vi "Acquire Data using 5772 without DRAM_sim2.vi"() -> ()   [LabVIEW 2011]
uses:
  <vilib>/Platform/TimedLoop/XDataNode/timing_clust.ctl
  <vilib>/Platform/TimedLoop/XDataNode/nitl_modes.ctl
  <vilib>/Platform/TimedLoop/XDataNode/wakeup.ctl
  <instrlib>/FlexRIO/Libraries/Acquisition Engine/FPGA/Implementation/Pack 8-I16 As U128.vi
  <instrlib>/FlexRIO/Libraries/Host Transfer/FPGA/Implementation/Write to Host-Bound Domain (128-bit to 64-bit).vi
  <vilib>/rvi/FIFO/Fifo_Resource/nirvififoEmulationSetSize.vi
  <vilib>/rvi/DataTransferAndStorage/Container/Common/niFpgaContainerGetUniqueNameForEmu.vi
  Channel Data/Data from Channel 0 and Channel 1.vi
  <instrlib>/FlexRIO/Libraries/Acquisition Engine/FPGA/Implementation/acqEngineNRecordStateMachine.vi
  <vilib>/Platform/TimedLoop/XDataNode/XDataNode.xnode
  <vilib>/rvi/DataTransferAndStorage/Container/XNode/niFpgaContainer.xnode
  <vilib>/rvi/FIFO/Fifo_Resource/nirvififoEmulationRead.vi
  <vilib>/rvi/FXPMathLib/basic elements/FxpDiscreteDelay/XNode/nifxpmath_DiscreteDelay.xnode
  <vilib>/rvi/FIFO/Fifo_Resource/nirvififoEmulationWrite.vi
  <vilib>/Platform/TimedLoop/XDataNode/XDNodeRunTimeDep.lvlib
  <vilib>/eio/EIONode/EIONode.xnode
  <instrlib>/FlexRIO/Libraries/Host Transfer/Host Transfer.lvlib
  <instrlib>/FlexRIO/Libraries/Acquisition Engine/Acquisition Engine.lvlib
  <vilib>/rvi/eio/common/nirviEmuTemplateMethod_errors.vi
panel:
  out "Trig[N-3]":bool
  out "Trig[N-2]":bool
  out "Trig[N-1]":bool
  out "Trig[N]":bool
  out "Q3":i16[](array[numeric])
  out "Q2":i16[](array[numeric])
  out "Q1":i16[](array[numeric])
  out "Channel 1":i16(graph)
  out "Channel 0":i16(graph)
  out "NumSamplestoHost":u32
  out "NumSamplesAcquired":u32
  out "Host FIFO Timed Out?":bool
  in  "Host Trigger":bool=TRUE
  in  "Trigger Type":T1(ring)=enum."Software Trigger"
  out "IO Module\\Initialization Done":bool
  in  "acq.Post Trig":u32=10
  in  "acq.Pre Trig":u32=2 min=2 step=1
  in  "acq.Record Count":u32=1
  in  "acq.Initiate":bool=TRUE
  # "Digitial Trigger Input:\nPXI_Trig0 or DIO 0 on CB Front Panel"
  # "Interactive Mode Instructions\n1) Run the Emulation Mode VI for Stimulus\n1) Click on acq.Initiate, First to False and Then to True\n2) Click on Host Trigger"
  # "Trigger Selection"
  # "Acquisition Engine"
  # "Status"
  # "Record Retrieval"
  # "Memory Configuration"
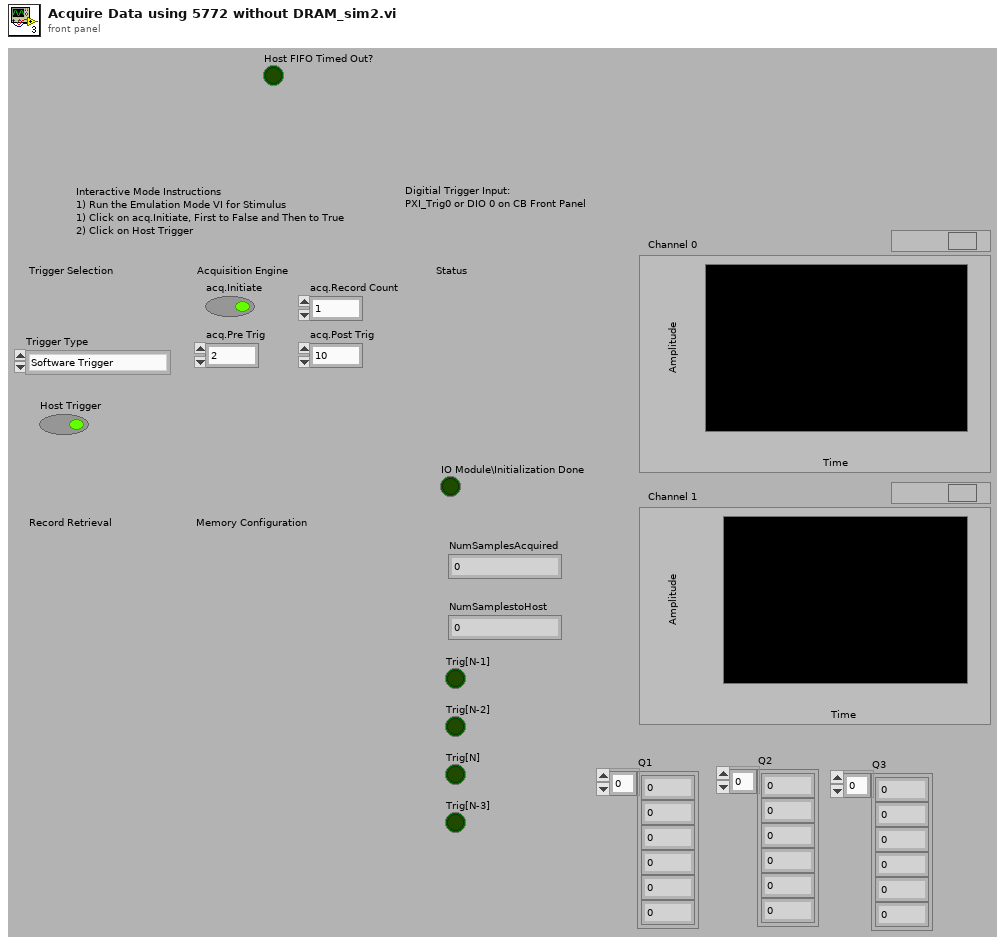
[diagram p1: front panel]
types:
  T1 = enum8{"Immediate Trigger", "Software Trigger", "External Digital Trigger", "Analog Trigger"}
  T2 = typedef "XDNodeRunTimeDep.lvlib/timing_clust.ctl" = cluster{"Expected End [f-1]":u64, "Actual End [f-1]":u64, "Finished Late? [f-1]":bool, "Expected End [i-1]":u64, "Actual End [i-1]":u64, "Finished Late? [i-1]":bool, "Expected Start [i]":u64, "Actual Start [i]":u64, "Expected Start [f]":u64, "Actual Start [f]":u64, "Source Name":string, "Structure Name":string, "Period":i64, "Deadline":i64, "Offset":i64, "Start":i64, "Priority":i32, "Timeout":i32, "Mode":T3, "Wakeup Reason":T4, "Error":errorcluster, "Source Type":string, "Secondary Source Type":string, "Global End Time":u64, "Global Start Time":u64, "Frame Duration":u64, "Iteration Duration":u64, "Assigned CPU":i32, "I/O Scan Engine Mode":u32}
  T3 = typedef "XDNodeRunTimeDep.lvlib/nitl_modes.ctl" = enum32{"No Change", "Process missed periods, maintain original phase", "Discard missed periods, maintain original phase", "Process missed periods, ignore original phase", "Discard missed periods, ignore original phase"}
  T4 = typedef "XDNodeRunTimeDep.lvlib/wakeup.ctl" = enum32{"Normal", "Aborted", "Asynchronous wakeup", "Timing source error", "Timed loop error", "Timeout"}
  T5 = typedef "acqEngineStates v1.ctl" = cluster{"Triggered":bool, "TrigArmed":bool, "RdyForArm":bool, "Reserved":bool}
  T6 = typedef "Memory.lvlib/U128.ctl" = u8[]
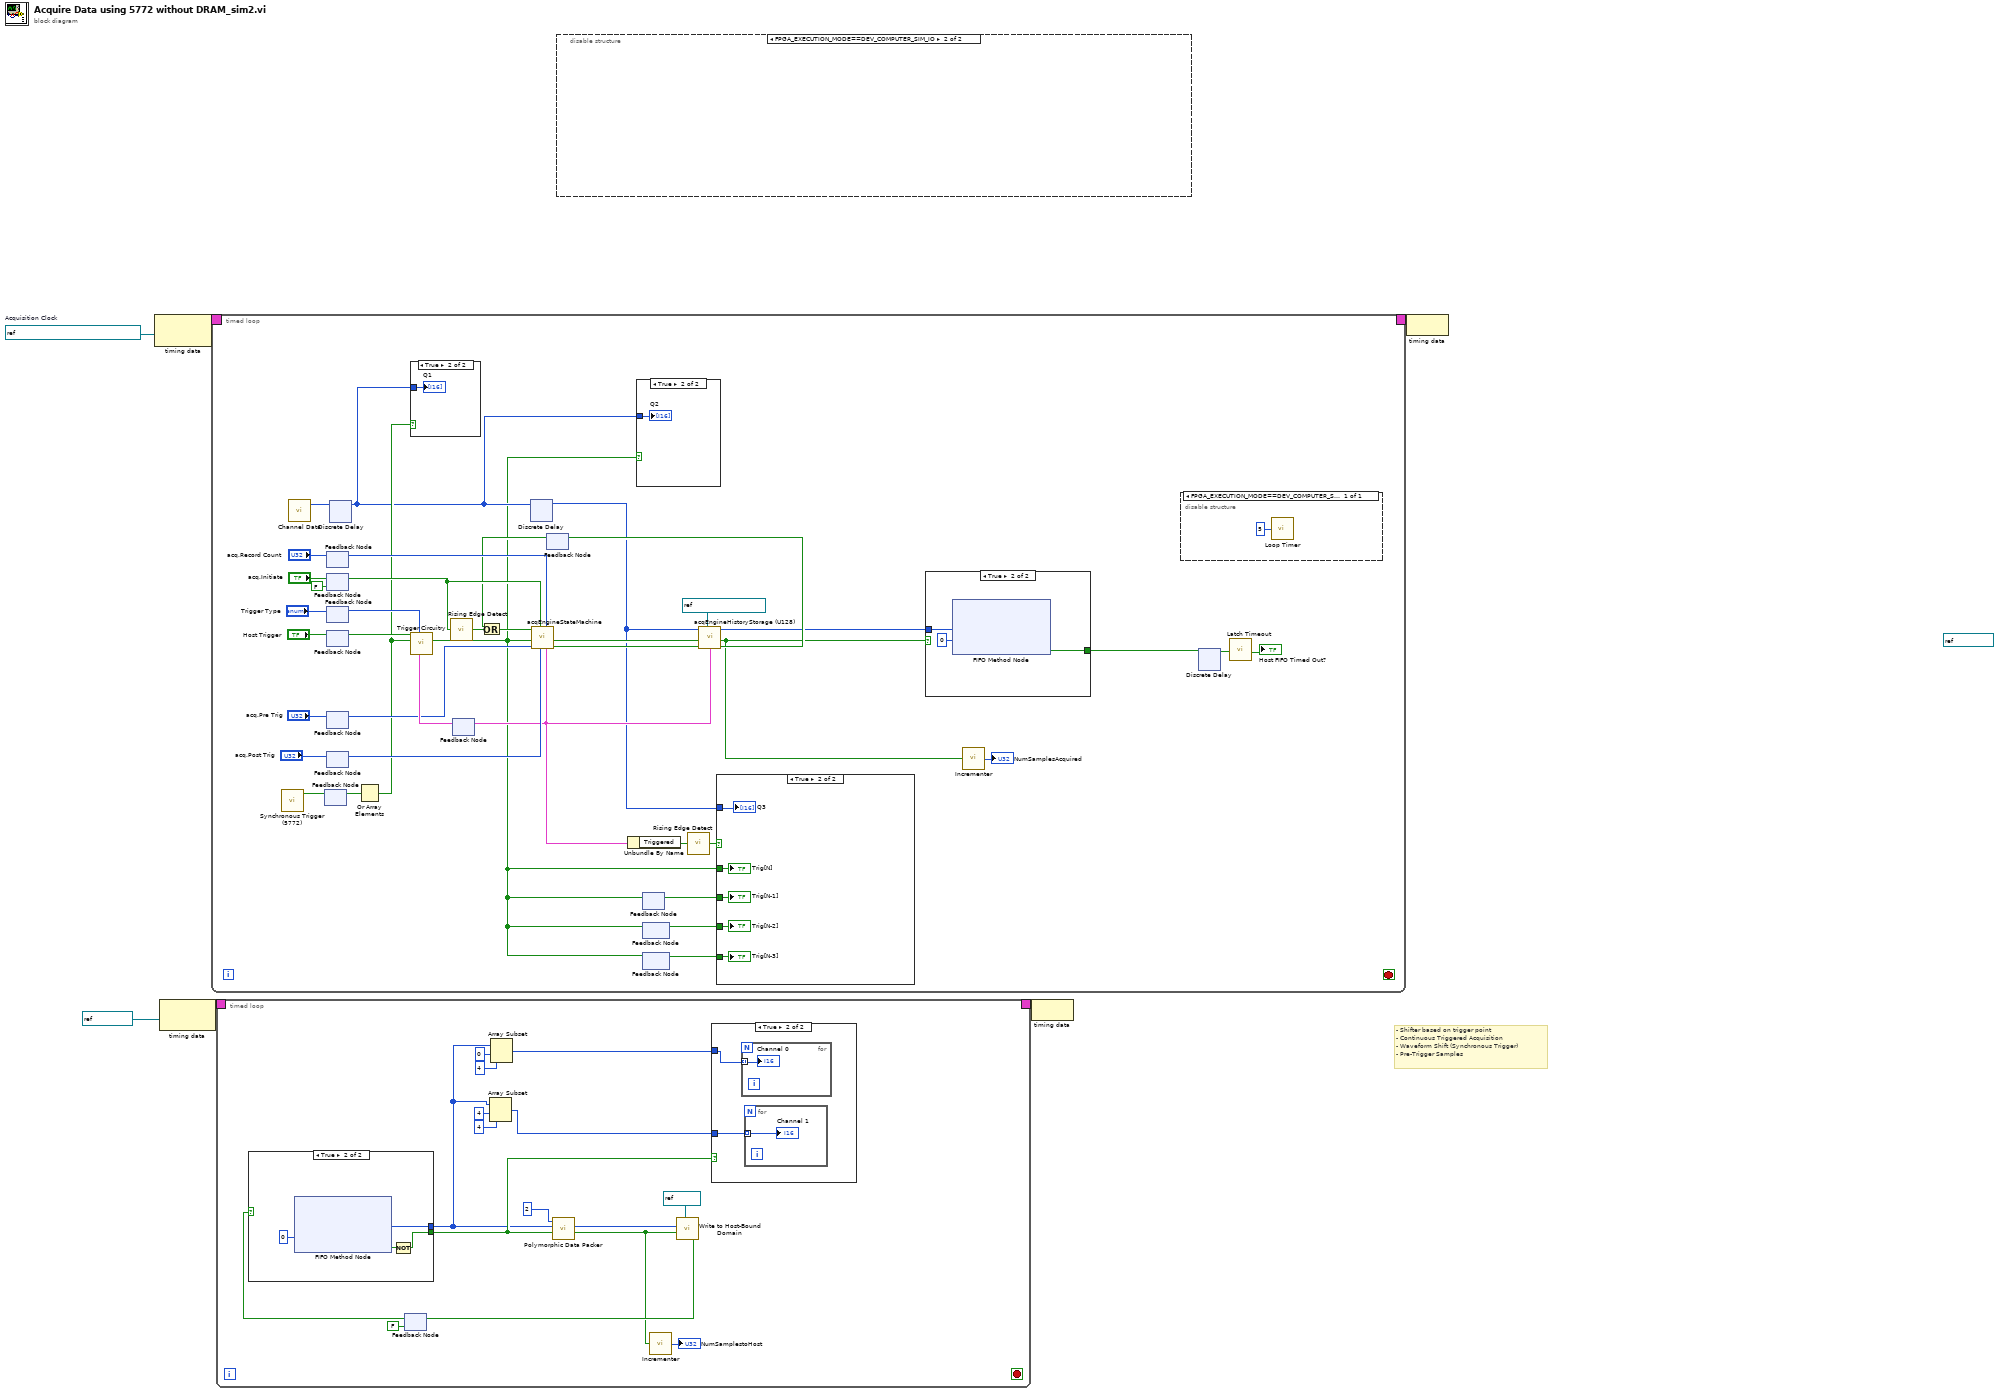
[diagram p0: block diagram]
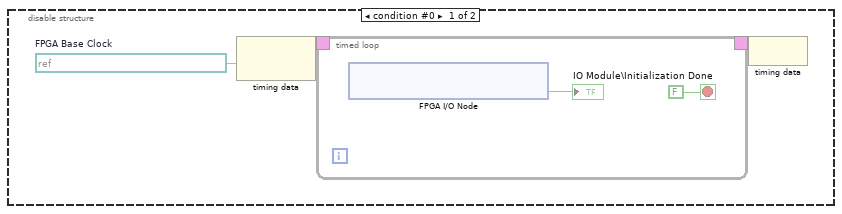
[diagram p2: hidden frame]
diagram:
  (unwired) refnum<k21> "To Host" ("FIFO In")
  w4 = refnum<k21> "IO Module Clock 0"  # Acquisition Clock
  # "- Shifter based on trigger point\n- Continuous Triggered Acquisition\n- Waveform Shift (Synchronous Trigger)\n- Pre-Trigger Samples"
  n1 = node-c288(w4) -> (w6:T2)
  n2 = node-c288(refnum<k21> "125MHz" ("Source Name")) -> (w3:T2)
  n3 = timed-loop {
    timing: w6 -> [_]
    timing-out: [_] -> w5
    stop <- _ stop-if-true
    n4 = call "Synchronous Trigger (5772).vi"() -> ("Trigger"=w22:bool[])  [unwired: 10 in, 1 out]
    n5 = call-poly "Channel Data.vi"() -> ("Channels Data"=w36:i16[])  [unwired: 11 in]
    n6 = feedback-in #1(w22) -> ()
    n7 = feedback #1() -> (w21:bool[])  [unwired: 1 in]
    n8 = feedback-in #2("acq.Record Count") -> ()
    n9 = feedback #2() -> (w40:u32)  [unwired: 1 in]
    n10 = feedback-in #3("acq.Initiate") -> ()
    n11 = feedback #3(FALSE ("acq.Initiate")) -> (w26:bool)
    n12 = feedback #4() -> (w38:T1)  [unwired: 1 in]
    n13 = feedback-in #4("Trigger Type") -> ()
    n14 = feedback-in #5("Host Trigger") -> ()
    n15 = feedback #5() -> (w37:bool)  [unwired: 1 in]
    n16 = feedback-in #6("acq.Pre Trig") -> ()
    n17 = feedback #6() -> (w35:u32)  [unwired: 1 in]
    n18 = feedback-in #7("acq.Post Trig") -> ()
    n19 = feedback #7() -> (w34:u32)  [unwired: 1 in]
    n20 = xnode "Discrete Delay"("D"=w36) -> ("Q"=w13:i16[])
    n21 = Or Array Elements(Boolean array=w21) -> (logical OR=w16:bool)
    n22 = case shown="True" w16 {
      tunnel: w13 -> [_ w53]
      frame False {
      }
      frame True {
        "Q1" <- w53
      }
    }
    n23 = call <userlib>:"Rising Edge Detect.vi"("signal"=w26) -> ("edge detected"=w23:bool)  [unwired: 14 in]
    n24 = feedback #8() -> (w42:T5)  [unwired: 1 in]
    n25 = call <userlib>:"Trigger Circuitry.vi"("State Machine State"=w42, "Trigger Type"=w38, "Digital Line Read"=w16, "Software Trigger from Host"=w37) -> ("Trigger Out"=w9:bool)  [unwired: 6 in, 1 out]
    n26 = xnode "Discrete Delay"("D"=w13) -> ("Q"=w12:i16[])
    n27 = feedback #9() -> (w24:bool)  [unwired: 1 in]
    n28 = Or(x=w24, y=w23) -> (x .or. y?=w25:bool)
    n29 = call-poly <instrlib>:"acqEngineStateMachine.vi"("acq.Record Count"=w40, "acq.Post Trig"=w34, "acq.Initiate"=w26, "acq.Pre Trig"=w35, "Trig"=w9, "StartTrig"=w25) -> ("PostTrigComplete"=w33:bool, "AcqInProgress"=w20:bool, "states"=w15:T5)  [unwired: 3 in]
    n30 = feedback-in #8(w15) -> ()
    n31 = Unbundle By Name(w15) -> ("Triggered"=w14:bool)
    n32 = case shown="True" w9 {
      tunnel: w13 -> [_ w52]
      frame False {
      }
      frame True {
        "Q2" <- w52
      }
    }
    n33 = feedback-in #10(w9) -> ()
    n34 = feedback #10() -> (w11:bool)  [unwired: 1 in]
    n35 = feedback #11() -> (w10:bool)  [unwired: 1 in]
    n36 = feedback-in #11(w9) -> ()
    n37 = feedback #12() -> (w8:bool)  [unwired: 1 in]
    n38 = feedback-in #12(w9) -> ()
    n39 = call <userlib>:"Rising Edge Detect.vi"("signal"=w14) -> ("edge detected"=w7:bool)  [unwired: 14 in]
    n40 = call "acqEngineHistoryStorage (U128).vi"("FIFO Out"=refnum<k21> "HistoryFIFOU128", "PostTrigComplete"=w33, "AcqInProgress"=w20, "states"=w15, "Input Data"=w12) -> ("flushed"=w27:bool, "valid"=w17:bool, "Output Data"=w18:i16[])  [unwired: 4 in]
    n41 = feedback-in #9(w27) -> ()
    n42 = case shown="True" w7 {
      tunnel: w12 -> [_ w51]
      tunnel: w9 -> [_ w50]
      tunnel: w11 -> [_ w49]
      tunnel: w10 -> [_ w48]
      tunnel: w8 -> [_ w47]
      frame False {
      }
      frame True {
        "Q3" <- w51
        "Trig[N]" <- w50
        "Trig[N-1]" <- w49
        "Trig[N-2]" <- w48
        "Trig[N-3]" <- w47
      }
    }
    n43 = case shown="True" w17 {
      tunnel: w18 -> [_ w57]
      tunnel: [_ w55] -> w29
      frame False {
      }
      frame True {
        n44 = xnode ("FIFO Method Node")("Element"=w57, "Timeout"=0) -> ("Timed Out?"=w55:bool)  [unwired: 1 in, 1 out]
      }
    }
    n45 = call <userlib>:"Incrementer.vi"("INC?"=w17) -> ("count"=→"NumSamplesAcquired":u32)  [unwired: 4 in]
    n46 = disable-structure shown="FPGA_EXECUTION_MODE==DEV_COMPUTER_SIM_IO, default" {
      frame condition #0 (active) {
        n47 = call "Loop Timer"("Count(mSec)"=u32 5) -> ()  [unwired: 1 out]
      }
    }
    n48 = xnode "Discrete Delay"("D"=w29) -> ("Q"=w30:bool)
    n49 = call <userlib>:"Latch Timeout.vi"("Timeout?"=w30) -> ("Ever Timed Out?"=→"Host FIFO Timed Out?":bool)  [unwired: 10 in]
  }
  n50 = timed-loop {
    timing: w3 -> [_]
    timing-out: [_] -> w2
    stop <- _ stop-if-true
    n51 = feedback #13(FALSE ("Ready For Input")) -> (w73:bool)
    n52 = case shown="True" w73 {
      tunnel: [_ w82] -> w61
      tunnel: [_ w80] -> w67
      frame False {
      }
      frame True {
        n53 = xnode ("FIFO Method Node")("Timeout"=0) -> ("Element"=w82:i16[], "Timed Out?"=w81:bool)  [unwired: 1 in, 1 out]
        n54 = Not(x=w81) -> (.not. x?=w80:bool)
      }
    }
    n55 = Array Subset(array=w61, index=4, length=4) -> (w60:i16[])
    n56 = Array Subset(array=w61, index=0, length=4) -> (w64:i16[])
    n57 = call-poly <instrlib>:"Polymorphic Data Packer.vi"("enable"=w67, "data"=w61, "Channels Per Unit"=u8 2) -> ("validOut"=w68:bool, "i16 as i128"=w69:T6)  [unwired: 4 in, 3 out]
    n58 = call <userlib>:"Incrementer.vi"("INC?"=w68) -> ("count"=→"NumSamplestoHost":u32)  [unwired: 4 in]
    n59 = call-poly <instrlib>:"Write to Host-Bound Domain.vi"("data"=w69, "valid"=w68, "FIFO Out"=refnum<k21> "FIFO") -> ("Ready For Input"=w74:bool)  [unwired: 4 in]
    n60 = feedback-in #13(w74) -> ()
    n61 = case shown="True" w67 {
      tunnel: w64 -> [_ w77]
      tunnel: w60 -> [_ w76]
      frame False {
      }
      frame True {
        n62 = for {
          tunnel: w77 -> [w79] mode=indexing
          "Channel 0" <- w79
        }
        n63 = for {
          tunnel: w76 -> [w78] mode=indexing
          "Channel 1" <- w78
        }
      }
    }
  }
  n64 = disable-structure shown="FPGA_EXECUTION_MODE==DEV_COMPUTER_SIM_IO" {
    frame condition #0 {
      w86 = refnum<k21> "40 MHz Onboard Clock"  # FPGA Base Clock
      n65 = node-c288(w86) -> (w88:T2)
      n66 = timed-loop {
        timing: w88 -> [_]
        timing-out: [_] -> w87
        stop <- FALSE stop-if-true
        n67 = xnode "FPGA I/O Node"() -> ("IO Module\\Initialization Done"=→"IO Module\\Initialization Done":bool)  [unwired: 1 in, 1 out]
      }
      n68 = node-c288(w87) -> ()
    }
    frame condition #1 (active) {
    }
  }
  n69 = node-c288(w2) -> ()
  n70 = node-c288(w5) -> ()
